vi "Toggle Menu Action.vi"(8 "error in (no error)":errorcluster, 10 "(T)Down (F) Up":bool, 11 "User Interface References":T1={"This VI"=refnum, "User Interace Plugin"=refnum, "UI Picture Container References"={"Header Image"=refnum, "Footer Image"=refnum}, "Sliding Menu XControl"=refnum, "Menu Container"=refnum, "UI Configuration Information"={"Space Between Buttons"=3, "Number of Buttons to Show"=6, "Header Image"=path "Images/Blue Background.bmp", "Footer Image"=path "Images/Blue Background.bmp"}, "Header Text"=refnum}) -> (0 "error out":errorcluster, 3 "User Interface References Out":T1={"This VI"=refnum, "User Interace Plugin"=refnum, "UI Picture Container References"={"Header Image"=refnum, "Footer Image"=refnum}, "Sliding Menu XControl"=refnum, "Menu Container"=refnum, "UI Configuration Information"={"Space Between Buttons"=3, "Number of Buttons to Show"=6, "Header Image"=path "Images/Blue Background.bmp", "Footer Image"=path "Images/Blue Background.bmp"}, "Header Text"=refnum})   [LabVIEW 2011]
uses:
  Main Type Definitions/User Interface Type Definitions.ctl
  Main Type Definitions/UI Picture Containers.ctl
  Sliding Menu/Sliding Menu Library/Sliding Menu xControl/Sliding Menu XControl.xctl
  User Interface/UI Control Definitions/UI Configuration Information.ctl
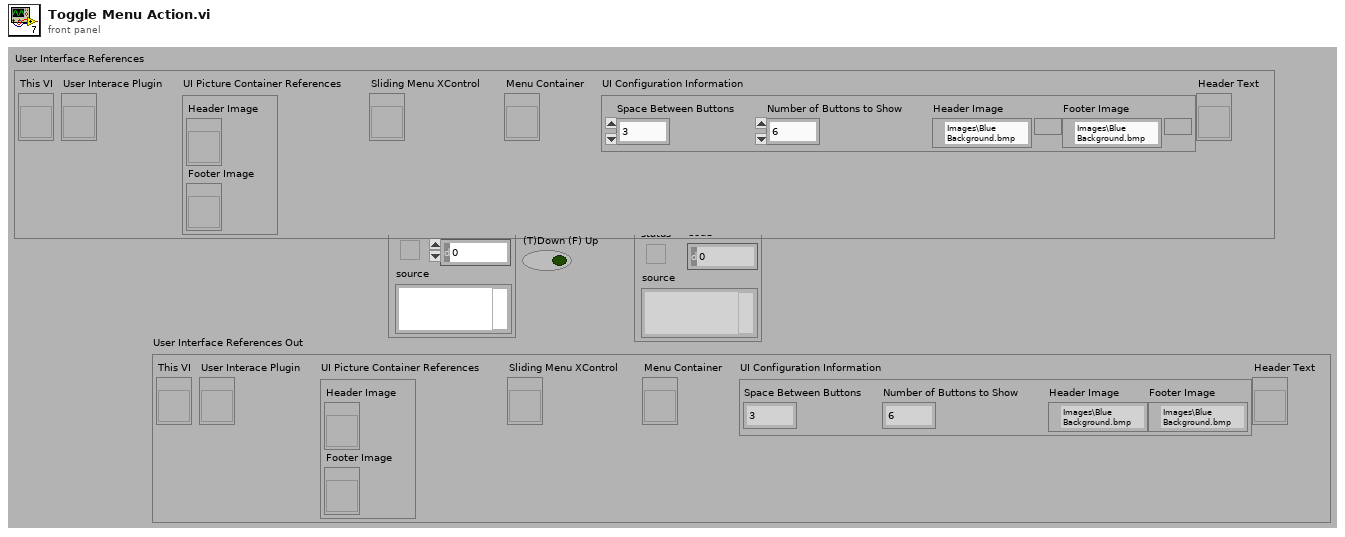
[diagram p1: front panel]
types:
  T1 = typedef "User Interface Type Definitions.ctl" = cluster{"This VI":refnum<vi>, "User Interace Plugin":refnum<vi>, "UI Picture Container References":T2, "Sliding Menu XControl":refnum<vi>, "Menu Container":refnum<vi>, "UI Configuration Information":T3, "Header Text":refnum<vi>}
  T2 = typedef "UI Picture Containers.ctl" = cluster{"Header Image":refnum<vi>, "Footer Image":refnum<vi>}
  T3 = typedef "UI Configuration Information.ctl" = cluster{"Space Between Buttons":i32, "Number of Buttons to Show":i32, "Header Image":path, "Footer Image":path}
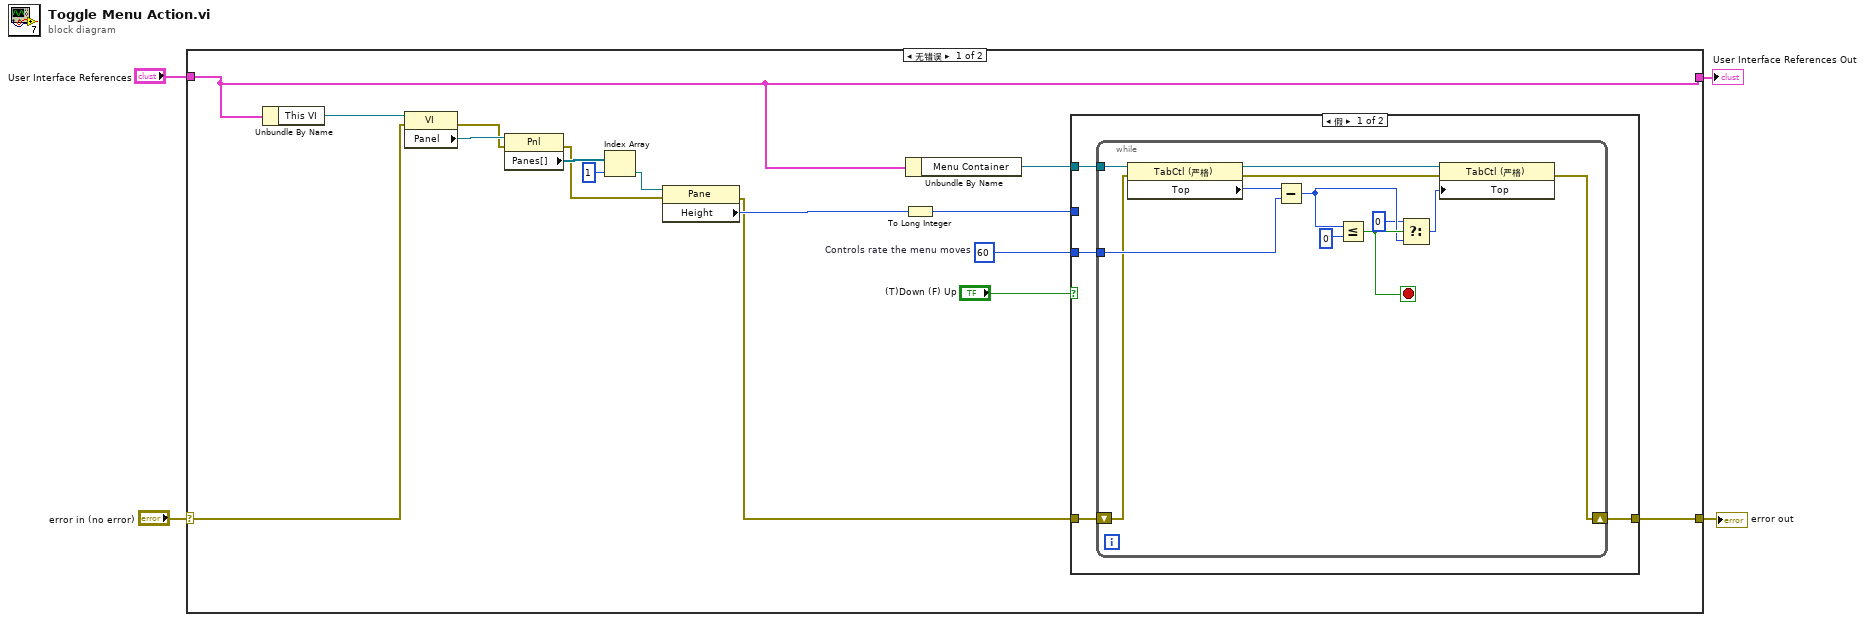
[diagram p0: block diagram]
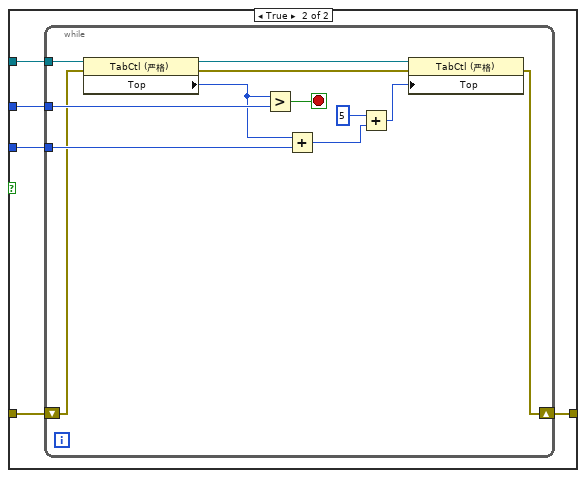
[diagram p2: hidden frame]
diagram:
  n1 = case shown="无错误" "error in (no error)" {
    selector: "error in (no error)" -> [w7 w55]
    tunnel: [w5 w55] -> w1
    tunnel: "User Interface References" -> [w13 w54]
    tunnel: [w13 w54] -> w4
    frame No Error {
      w8 = 60  # Controls rate the menu moves
      n2 = Unbundle By Name(w13) -> ("This VI"=w20:refnum<vi>)
      n3 = property class="VI"(reference=w20, error in=w7) -> (error out=w14:errorcluster, "Panel"=w19:refnum<vi>)  [unwired: 1 out]
      n4 = property class="Pnl"(reference=w19, error in=w14) -> (error out=w15:errorcluster, "Panes[]"=w18:refnum<vi>[])  [unwired: 1 out]
      n5 = Index Array(array=w18, index=1) -> (element=w16:refnum<vi>)
      n6 = property class="Pane"(reference=w16, error in=w15) -> (error out=w6:errorcluster, "Height"=w11:u32)  [unwired: 1 out]
      n7 = To Long Integer(number=w11) -> (32bit integer=w10:i32)
      n8 = Unbundle By Name(w13) -> ("Menu Container"=w12:refnum<vi>)
      n9 = case shown="假" "(T)Down (F) Up" {
        tunnel: w12 -> [w24 w41]
        tunnel: w10 -> [_ w40]
        tunnel: w8 -> [w23 w39]
        tunnel: w6 -> [w22 w38]
        tunnel: [w21 w37] -> w5
        frame False {
          n10 = while {
            tunnel: w24 -> [w36]
            tunnel: w23 -> [w28]
            shift-right: [w26] -> w21
            shift-left: w22 -> [w27]
            stop <- w32 stop-if-true
            n11 = property class="TabCtl (严格)"(reference=w36, error in=w27) -> (reference out=w34:refnum<vi>, error out=w25:errorcluster, "Top"=w33:i32)
            n12 = Subtract(x=w33, y=w28) -> (x-y=w31:i32)
            n13 = Less Or Equal?(x=w31, y=0) -> (x <= y?=w32:bool)
            n14 = Select(t=0, s=w32, f=w31) -> (s? t:f=w30:i32)
            n15 = property class="TabCtl (严格)"(reference=w34, error in=w25, "Top"=w30) -> (error out=w26:errorcluster)  [unwired: 1 out]
          }
        }
        frame True {
          n16 = while {
            tunnel: w40 -> [w50]
            tunnel: w41 -> [w53]
            tunnel: w39 -> [w45]
            shift-right: [w42] -> w37
            shift-left: w38 -> [w44]
            stop <- w52 stop-if-true
            n17 = property class="TabCtl (严格)"(reference=w53, error in=w44) -> (reference out=w51:refnum<vi>, error out=w43:errorcluster, "Top"=w49:i32)
            n18 = Greater?(x=w49, y=w50) -> (0:w52:bool)
            n19 = Add(x=w49, y=w45) -> (x+y=w48:i32)
            n20 = Add(x=5, y=w48) -> (x+y=w47:i32)
            n21 = property class="TabCtl (严格)"(reference=w51, error in=w43, "Top"=w47) -> (error out=w42:errorcluster)  [unwired: 1 out]
          }
        }
      }
    }
    frame Error {
    }
  }
  "error out" <- w1
  "User Interface References Out" <- w4
